vi "DeleteTileFromRiver.vi"(10 "Player":T1) -> (1 "DeletedTile":u16(ring), 2 "NewPlayer":T1)   [LabVIEW 2025]
uses:
  Controls/Player.ctl
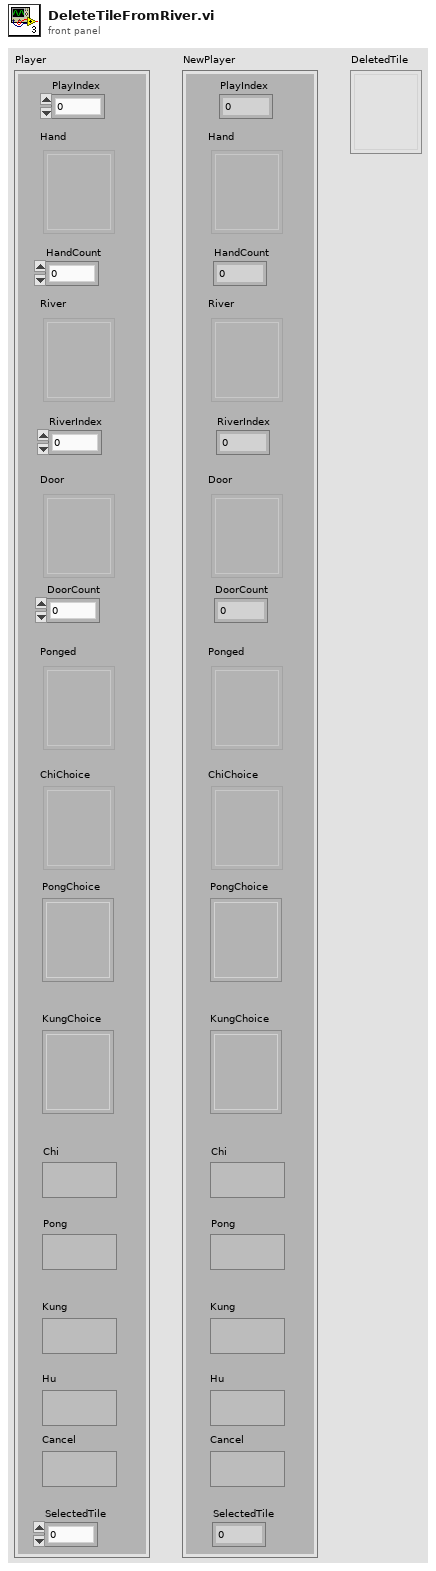
[diagram p1: front panel]
types:
  T1 = typedef "Player.ctl" = cluster{"PlayIndex":u16, "Hand":u16[], "HandCount":u16, "RiverIndex":u16, "Door":u16[], "DoorCount":u16, "Ponged":u16[], "ChiChoice":u16[][], "River":u16[][], "Chi":bool, "Pong":bool, "Kung":bool, "Hu":bool, "Cancel":bool, "PongChoice":u16, "KungChoice":u16, "SelectedTile":i16}
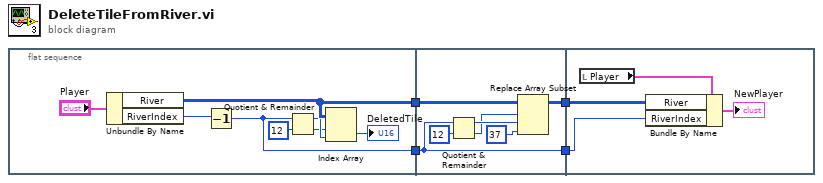
[diagram p0: block diagram]
diagram:
  n1 = flat-sequence {
    tunnel: [w5] -> w4
    tunnel: [w9] -> w3
    tunnel: w4 -> [w17]
    tunnel: w3 -> [w14]
    tunnel: [w17] -> w2
    tunnel: [w13] -> w1
    tunnel: w2 -> [w20]
    tunnel: w1 -> [w22]
    frame #0 {
      n2 = Unbundle By Name("Player") -> ("River"=w9:u16[][], "RiverIndex"=w6:u16)
      n3 = Decrement(x=w6) -> (x-1=w5:u16)
      n4 = Quotient & Remainder(x=w5, y=12) -> (x-y*floor(x/y)=w8:i32, floor(x/y)=w7:i32)
      n5 = Index Array(array=w9, index (row)=w7, index (col)=w8) -> (element=→"DeletedTile":u16)
    }
    frame #1 {
      n6 = Quotient & Remainder(x=w17, y=12) -> (x-y*floor(x/y)=w16:i32, floor(x/y)=w15:i32)
      n7 = Replace Array Subset(array=w14, new element=37, index (row)=w15, index (col)=w16) -> (w13:u16[][])
    }
    frame #2 {
      n8 = local read "Player"() -> (w21:T1)
      n9 = Bundle By Name(cluster=w21, "River"=w22, "RiverIndex"=w20) -> (→"NewPlayer":T1)
    }
  }
